vi "assembly_result_table_I_cal.vi"(8 "error_in":errorcluster, 10 "result":dbl[][](array[numeric]), 11 "I_control_values":dbl[](array[numeric])) -> (0 "error_out":errorcluster, 3 "result_table":dbl[][](array[numeric]))   [LabVIEW 2017]
panel:
  out "abs":dbl[][](array[numeric])
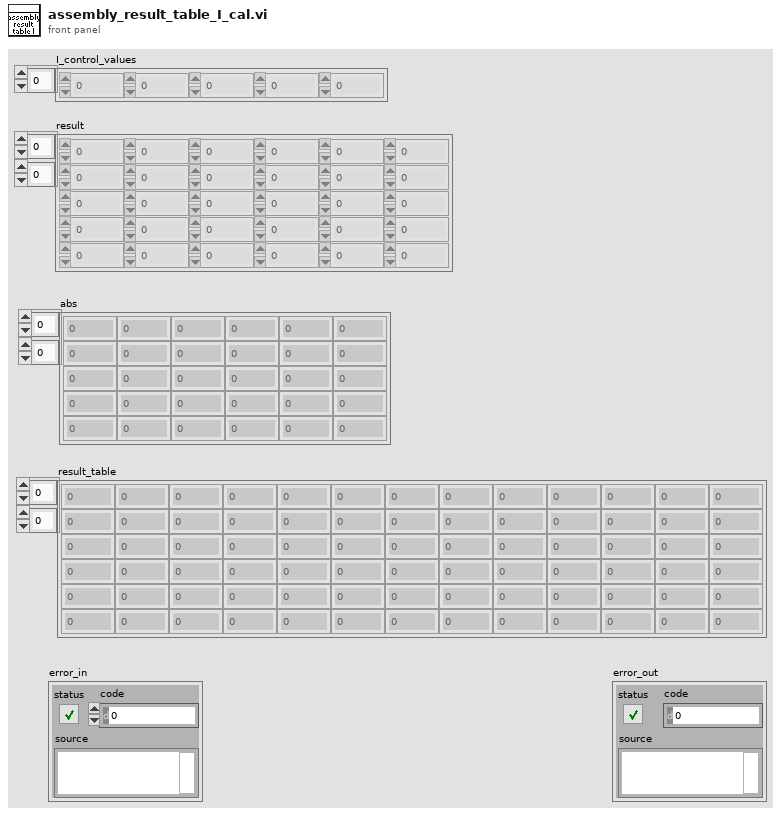
[diagram p1: front panel]
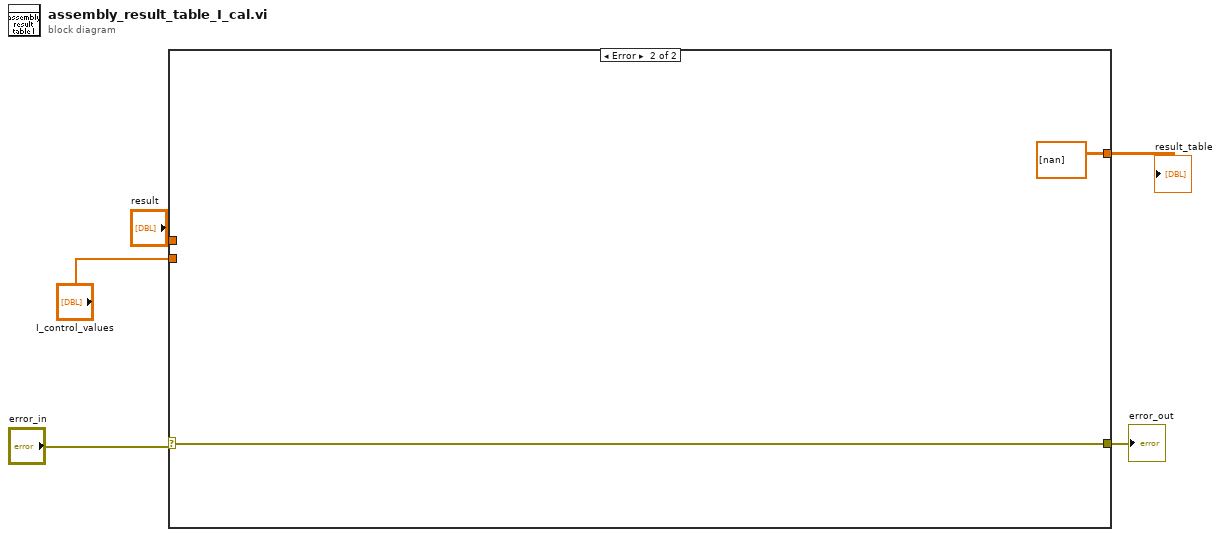
[diagram p0: block diagram]
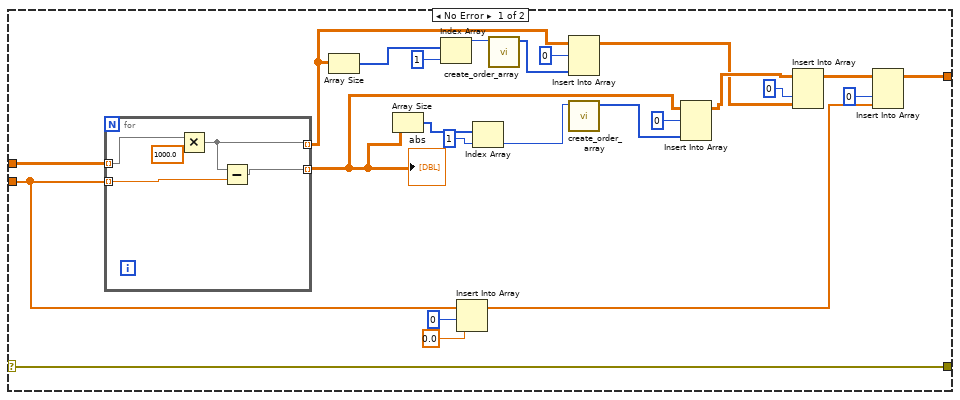
[diagram p2: hidden frame]
diagram:
  n1 = case shown="Error" "error_in" {
    selector: "error_in" -> [w6 w36]
    tunnel: "result" -> [w22 _]
    tunnel: [w14 dbl[][] [[nan]]] -> w4
    tunnel: "I_control_values" -> [w13 _]
    tunnel: [w6 w36] -> w2
    frame No Error {
      n2 = for {
        tunnel: w22 -> [w33] mode=indexing
        tunnel: w13 -> [w32] mode=indexing
        tunnel: [w31] -> w18 mode=indexing
        tunnel: [w30] -> w7 mode=indexing
        n3 = Multiply(x=w33, y=1000.0) -> (x*y=w30:dbl[])
        n4 = Subtract(x=w30, y=w32) -> (x-y=w31:dbl[])
      }
      "abs" <- w18
      n5 = Array Size(array=w7) -> (size(s)=w26:i32[])
      n6 = Array Size(array=w18) -> (size(s)=w29:i32[])
      n7 = Index Array(array=w26, index=1) -> (element=w24:i32)
      n8 = Insert Into Array(array=w13, index=0, new element=0.0 ("new element/subarray")) -> (w12:dbl[])
      n9 = Index Array(array=w29, index=1) -> (element=w25:i32)
      n10 = call "create_order_array.vi"("Numeric"=w24) -> ("Array"=w23:i32[])  [unwired: 10 in]
      n11 = Insert Into Array(array=w7, index (row)=0, new element=w23) -> (w8:dbl[][])  [unwired: 1 in]
      n12 = call "create_order_array.vi"("Numeric"=w25) -> ("Array"=w19:i32[])  [unwired: 10 in]
      n13 = Insert Into Array(array=w18, index (row)=0, new element=w19) -> (w9:dbl[][])  [unwired: 1 in]
      n14 = Insert Into Array(array=w9, index (col)=0 ("index (row)"), new element=w8) -> (w16:dbl[][])  [unwired: 1 in]
      n15 = Insert Into Array(array=w16, index (col)=0 ("disabled index (col)"), new element=w12) -> (w14:dbl[][])  [unwired: 1 in]
    }
    frame Error {
    }
  }
  "result_table" <- w4
  "error_out" <- w2
